vi "SeCrTs-Continuous or cummulative DI.vi"(8 "DI   data":bool[](array[boolean]), 9 "DI Channels Name":string[](array[string]), 10 "CDT":dbl, 11 "output cluster":T1) -> (2 "Failure case Seq":string, 3 "In Range":string)   [LabVIEW 2022 SP3]
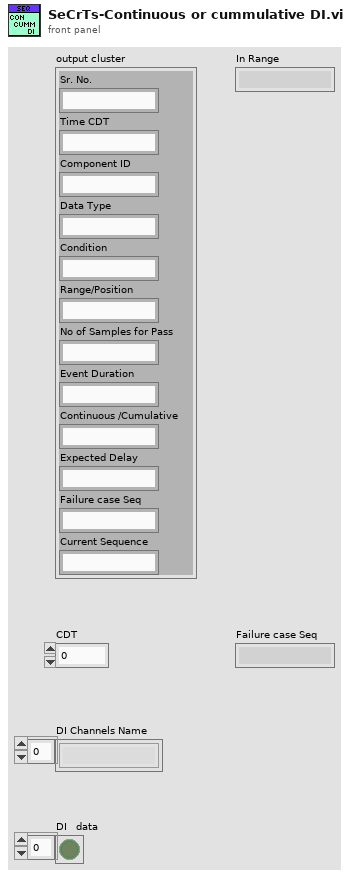
[diagram p1: front panel]
types:
  T1 = cluster{"Sr. No.":string, "Time CDT":string, "Component ID":string, "Data Type":string, "Condition":string, "Range/Position":string, "No of Samples for Pass":string, "Event Duration":string, "Continuous /Cumulative":string, "Expected Delay":string, "Failure case Seq":string, "Current Sequence":string}
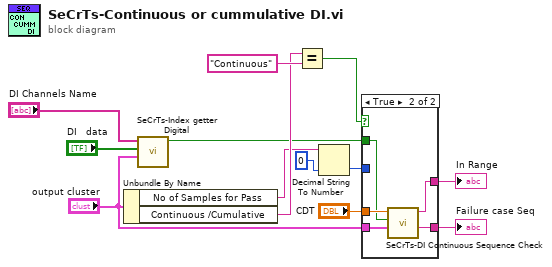
[diagram p0: block diagram]
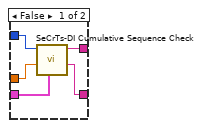
[diagram p2: hidden frame]
diagram:
  n1 = Unbundle By Name("output cluster") -> ("No of Samples for Pass"=w1:string, "Continuous /Cumulative"=w7:string)
  n2 = call "SeCrTs-Index getter  Digital.vi"("output cluster"="output cluster", "DI Y  data"="DI   data", "DI Channels Name"="DI Channels Name") -> ("Digital data"=w6:bool)  [unwired: 8 in]
  n3 = Equal?(x=w7, y="Continuous") -> (x = y?=w9:bool)
  n4 = Decimal String To Number(string=w1, default (0L)=0) -> (number=w11:i32)  [unwired: 1 in, 1 out]
  n5 = case shown="True" w9 {
    tunnel: w6 -> [_ w20]
    tunnel: "output cluster" -> [w16 w22]
    tunnel: w11 -> [w18 _]
    tunnel: [w15 w21] -> w5
    tunnel: "CDT" -> [w17 w23]
    tunnel: [w14 w19] -> w2
    frame False {
      n6 = call "SeCrTs-DI Cumulative Sequence Check.vi"("output cluster"=w16, "CDT"=w17, "Numeric 2"=w18) -> ("Failure case Seq"=w14:string, "String"=w15:string)  [unwired: 6 in, 1 out]
    }
    frame True {
      n7 = call "SeCrTs-DI Continuous Sequence Check.vi"("output cluster"=w22, "DI"=w20, "CDT"=w23) -> ("Failure case Seq"=w19:string, "In Range"=w21:string)  [unwired: 6 in, 1 out]
    }
  }
  "In Range" <- w5
  "Failure case Seq" <- w2
